vi "cut_initial_picture.vi"(0 "picture":picture) -> (4 "new":u32[][](array[numeric]))   [LabVIEW 2015]
uses:
  <vilib>/imath/engines/lvmath2/RunTimeEngine/RangeToken/NIMS_Range_R2 - Integer.vi
  <instcachedir>/0/NIMS_Range_R2 - Integer_396D5D4FB869421F9245109A0975AD54.lvgen/NIMS_Range_R2 - Integer_396D5D4FB869421F9245109A0975AD54_000.vi
  <vilib>/imath/engines/lvmath2/RunTimeEngine/CommandStatement/MC_CommandStatement_break.vi
  <vilib>/imath/engines/lvmath2/RunTimeSupport/NIMS_Error if Not Equal.vi
  <instcachedir>/0/NIMS_Error if Not Equal_7F0D61CE56BF44979916ECA34C78675F.lvgen/NIMS_Error if Not Equal_7F0D61CE56BF44979916ECA34C78675F_000.vi
  <vilib>/imath/engines/lvmath2/RunTimeEngine/IndexRead/NIMS M(S,S).vi
  <instcachedir>/0/NIMS M(S,S)_AC51E74150A542F7991B9634C66F3096.lvgen/NIMS M(S,S)_AC51E74150A542F7991B9634C66F3096_002.vi
  <vilib>/imath/engines/lvmath2/RunTimeEngine/IndexReplace/NIMS M(S,S)=S.vi
  <instcachedir>/0/NIMS M(S,S)=S_72298AC072A24B679F5E0C14DB2DD503.lvgen/NIMS M(S,S)=S_72298AC072A24B679F5E0C14DB2DD503_003.vi
  <vilib>/imath/engines/lvmath2/RunTimeEngine/ErrorHandling/NIMS_Create Error From Enums.vi
  <vilib>/imath/engines/lvmath2/RunTimeEngine/NodeEndStatement/NIMS_NodeEndStatement_Output.vi
  <instcachedir>/0/NIMS_NodeEndStatement_Output_53EC0D466D134D7ABD903AC30B43404B.lvgen/NIMS_NodeEndStatement_Output_53EC0D466D134D7ABD903AC30B43404B_016.vi
  <instcachedir>/0/NIMS_NodeEndStatement_Output_53EC0D466D134D7ABD903AC30B43404B.lvgen/NIMS_NodeEndStatement_Output_53EC0D466D134D7ABD903AC30B43404B_010.vi
  <vilib>/imath/engines/lvmath2/RunTimeEngine/ErrorHandling/NIMS_Finalize Error.vi
  <vilib>/picture/picture.llb/Draw True-Color Pixmap.vi
panel:
  out "new picture":picture
  out "24-bit pixmap":u32[][](array[numeric]) format="%x"
  out "x":i32
  out "element 2":i32
  out "element":i32
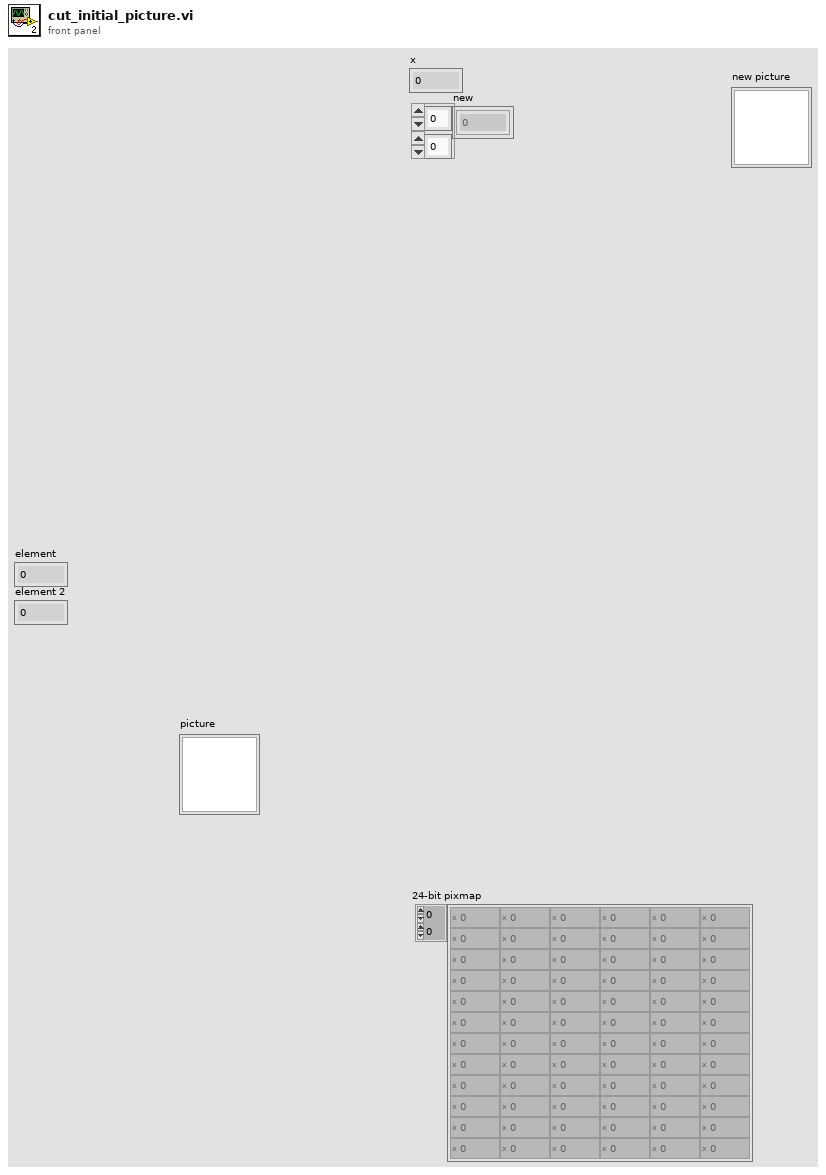
[diagram p1: front panel]
types:
  T1 = typedef "imagedata.ctl" = cluster{"image type":i32, "image depth":i32, "image":u8[], "mask":u8[], "colors":u32[], "Rectangle":cluster{"left":i16, "top":i16, "right":i16, "bottom":i16}}
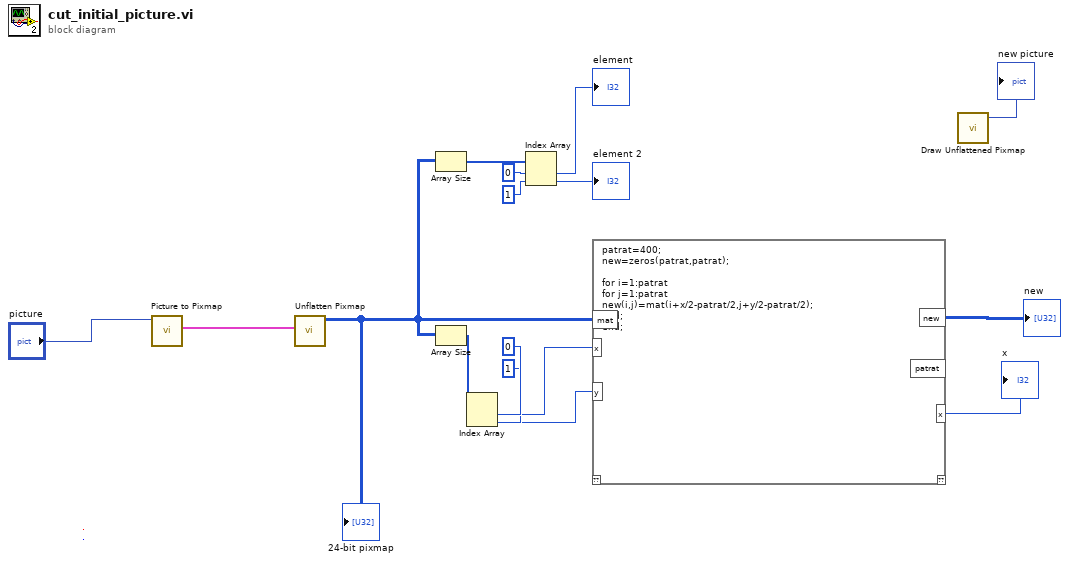
[diagram p0: block diagram]
diagram:
  n1 = call <vilib>:"Picture to Pixmap.vi"("picture"="picture") -> ("image data"=w5:T1)  [unwired: 9 in, 1 out]
  n2 = call <vilib>:"Unflatten Pixmap.vi"("image data"=w5) -> ("24-bit pixmap"=w3:u32[][])  [unwired: 4 in, 6 out]
  "24-bit pixmap" <- w3
  n3 = Array Size(array=w3) -> (size(s)=w16:i32[])
  n4 = Array Size(array=w3) -> (size(s)=w11:i32[])
  n5 = Index Array(array=w11, index #1=0 ("index"), index #2=1 ("index")) -> (element #1=w8:i32, element #2=w7:i32)
  n6 = Index Array(array=w16, index #1=0 ("index"), index #2=1 ("index")) -> (element #1=→"element":i32, element #2=→"element 2":i32)
  n7 = mathscript code="patrat=400;\nnew=zeros(patrat,patrat);\n\nfor i=1:patrat\nfor j=1:patrat\nnew(i,j)=mat(i+x/2-patrat/2,j+y/2-patrat/2);\nend;\nend;"("mat"=w3, "x"=w8, "y"=w7) -> ("new"=→"new":u32[][], "x"=→"x":i32)  [unwired: 1 in, 2 out]
  n8 = call-poly <vilib>:"Draw Unflattened Pixmap.vi"() -> ("new picture"=→"new picture":picture)  [unwired: 9 in]
